vi "float_precision.vi"(0 "input":dbl=22.2826 format="%#.12f", 1 "precision":i32=3) -> (2 "output":dbl=22.2826 format="%#.12f")   [LabVIEW 2016]
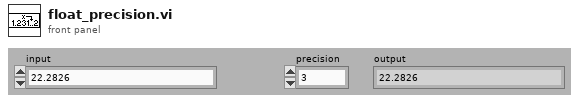
[diagram p1: front panel]
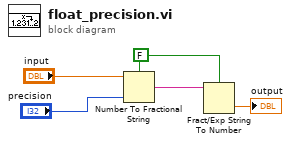
[diagram p0: block diagram]
diagram:
  w2 = FALSE ("use system decimal point (T)")
  n1 = Number To Fractional String(use system decimal point (T)=w2, number="input", precision (6)="precision") -> (F-format string=w3:string)  [unwired: 1 in]
  n2 = Fract/Exp String To Number(use system decimal point (T)=w2, string=w3) -> (number=→"output":dbl)  [unwired: 2 in, 1 out]
